vi "Close.vi"(8 "error in (no error)":errorcluster, 11 "HAL GOOP4:Series Base in":refnum<class "Series Base.lvclass">) -> (0 "error out":errorcluster, 3 "HAL GOOP4:Series Base out":refnum<class "Series Base.lvclass">)   [LabVIEW 2023, in "HAL GOOP4.lvlib" / "Series Base.lvclass"]
uses:
  Series Base.lvclass
  Series Base.lvclass/Series Base.ctl
  Measure and Stimulus Subsystems/Measure and Stimulus Subsystems.lvclass
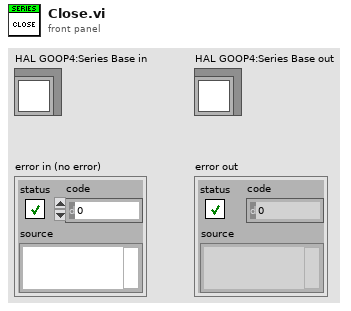
[diagram p1: front panel]
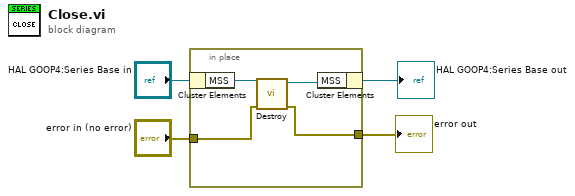
[diagram p0: block diagram]
diagram:
  n1 = in-place "In Place Element Structure" {
    in-place-border: "error in (no error)" -> [w6]
    in-place-border: [w5] -> w1
    n2 = in-place-cluster #1("HAL GOOP4:Series Base in") -> ("MSS"=w8:refnum<class "Measure and Stimulus Subsystems.lvclass">)
    n3 = call "Destroy.vi"("Error In"=w6, "reference in"=w8) -> ("Error Out"=w5:errorcluster, "reference out"=w7:refnum<class "Measure and Stimulus Subsystems.lvclass">)  [unwired: 8 in]
    n4 = in-place-cluster #1("MSS"=w7) -> (→"HAL GOOP4:Series Base out":refnum<class "Series Base.lvclass">)
  }
  "error out" <- w1
